vi "Configure Measurement (Transient).vi"(0 "VISA resource name":refnum<visa-resource-name>, 1 "Phase Reference (1E9 Hz)":dbl=1000000000.0 format="%^#_9g", 2 "Wideband Max Frequency (1.20E9 Hz)":dbl=1200000000.0 format="%^#_9g", 5 "Maximum Input Level (0 dBm)":dbl format="%^#_9g", 7 "Frequency Range (1: 25.6 MHz)":u16(ring)=1 format="%^#_9g" items=["80 MHz", "25.6 MHz", "1.6 MHz", "200 kHz", "25 kHz", "3.125 kHz"], 9 "Target Frequency (1E9 Hz)":dbl=1000000000.0 format="%^#_9g", 11 "error in (no error)":errorcluster, 12 "Phase Reference Offset (0 Hz)":dbl format="%^#_9g") -> (4 "VISA resource name out":refnum<visa-resource-name>, 15 "error out":errorcluster)   [LabVIEW 2011, in "Agilent E5052X.lvlib"]
doc: "Configures the instrument to take Transient measurements.\n\n<b>Note: </b> \n\n\"Configure Measurement Characteristics(Transient)\" VI must be called before calling this VI."
uses:
  Agilent E5052X.lvlib
panel:
  # "Narrowband Trace Settings"
  # "Wideband Trace Settings"
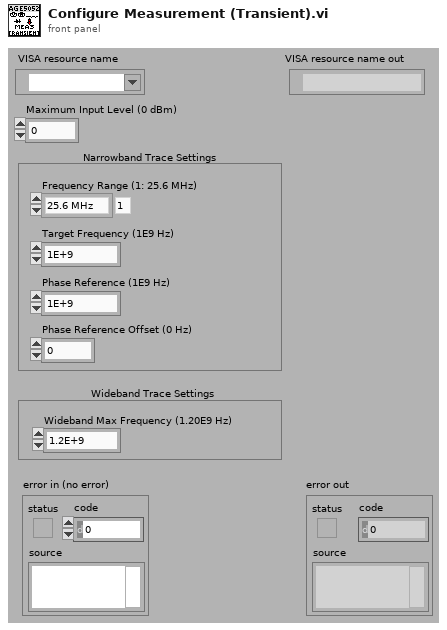
[diagram p1: front panel]
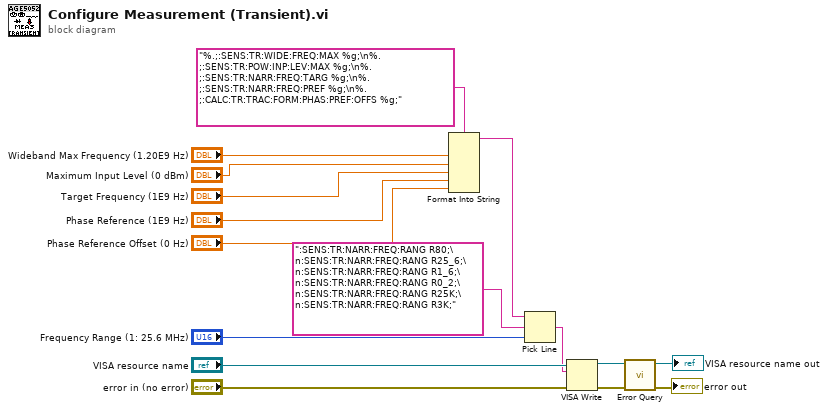
[diagram p0: block diagram]
diagram:
  n1 = Format Into String(format string="%.;:SENS:TR:WIDE:FREQ:MAX %g;\n%.;:SENS:TR:POW:INP:LEV:MAX %g;\n%.;:SENS:TR:NARR:FREQ:TARG %g;\n%.;:SENS:TR:NARR:FREQ:PREF %g;\n%.;:CALC:TR:TRAC:FORM:PHAS:PREF:OFFS %g;", "Wideband Max Frequency (1.20E9 Hz)", "Maximum Input Level (0 dBm)", "Target Frequency (1E9 Hz)", "Phase Reference (1E9 Hz)", "Phase Reference Offset (0 Hz)") -> (resulting string=w3:string)  [unwired: 2 in, 1 out]
  n2 = Pick Line(string ("")=w3, multi-line string=":SENS:TR:NARR:FREQ:RANG R80;\n:SENS:TR:NARR:FREQ:RANG R25_6;\n:SENS:TR:NARR:FREQ:RANG R1_6;\n:SENS:TR:NARR:FREQ:RANG R0_2;\n:SENS:TR:NARR:FREQ:RANG R25K;\n:SENS:TR:NARR:FREQ:RANG R3K;", line index="Frequency Range (1: 25.6 MHz)") -> (output string=w1:string)
  n3 = VISA Write(VISA resource name="VISA resource name", write buffer=w1, error in (no error)="error in (no error)") -> (VISA resource name out=w6:refnum<visa-resource-name>, error out=w5:errorcluster)  [unwired: 1 out]
  n4 = call "Error Query.vi"("error in (no error)"=w5, "VISA resource name"=w6) -> ("error out"=→"error out":errorcluster, "VISA resource name out"=→"VISA resource name out":refnum<visa-resource-name>)  [unwired: 6 in, 2 out]
